vi "lowgoalshoot.vi"(7 "Description":string, 8 "Command Info In":T1, 10 "Numeric":dbl, 11 "Setpoint":dbl) -> (0 "Command Info Out":T1)   [LabVIEW 2015]
uses:
  <vilib>/Rock Robotics/WPI/Framework/Command Status Info.ctl
  <vilib>/Rock Robotics/WPI/Framework/Completion Status.ctl
  <vilib>/Rock Robotics/WPI/Framework/Completion Notifier.ctl
  Implementation/intake Setpoints.ctl
  Implementation/intake Operations.ctl
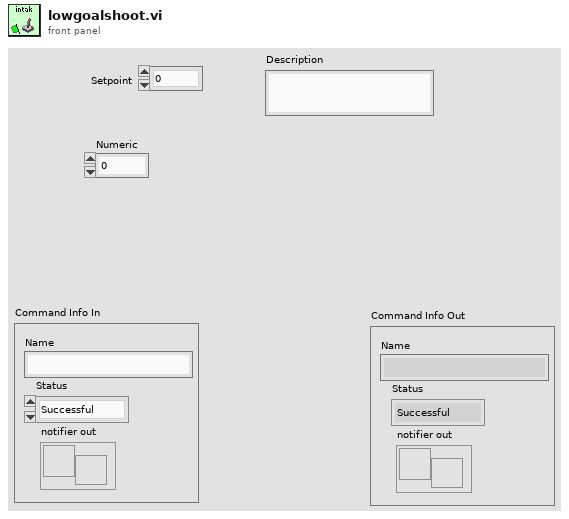
[diagram p1: front panel]
types:
  T1 = typedef "Command Status Info.ctl" = cluster{"Name":string, "Status":T2, "notifier out":T3}
  T2 = typedef "Completion Status.ctl" = enum16{"Successful", "Aborted", "Incomplete"}
  T3 = typedef "Completion Notifier.ctl" = refnum<notifier>
  T4 = typedef "intake Setpoints.ctl" = cluster{"Operation":T5, "Setpoint":dbl, "Duration":dbl, "up/down":dbl, "E-STOP":dbl, "Low goal?":dbl}
  T5 = typedef "intake Operations.ctl" = enum16{"Reserve", "Read Current", "Low Goal", "Shoot with intake", "down nd moving", "move up/down without moter moving", "move motor with out mving up/down", "extend and reverse"}
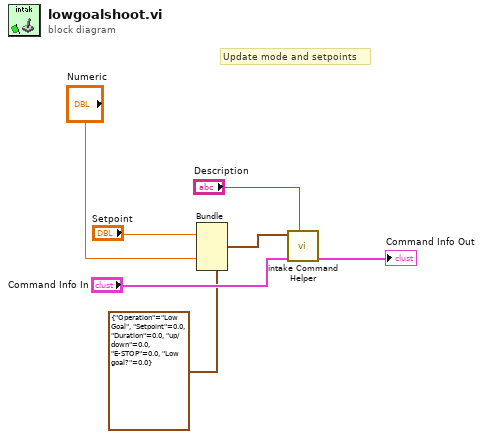
[diagram p0: block diagram]
diagram:
  # "Update mode and setpoints"
  n1 = Bundle(cluster=T4 {"Operation"=enum."Low Goal", "Setpoint"=0.0, "Duration"=0.0, "up/down"=0.0, "E-STOP"=0.0, "Low goal?"=0.0} ("SubSystem Data"), "Setpoint"="Setpoint", "E-STOP"="Numeric") -> (w2:T4)  [unwired: 4 in]
  n2 = call "intake Command Helper.vi"("Description"="Description", "Command Info In"="Command Info In", "SubSystem Data"=w2) -> ("Command Info Out"=→"Command Info Out":T1)  [unwired: 7 in, 1 out]
